vi "add channel to active array_wwarning.vi"(1 "line to add":u32, 2 "line array in":u32[](array[numeric])) -> (0 "line array out":u32[](array[numeric]))   [LabVIEW 2013]
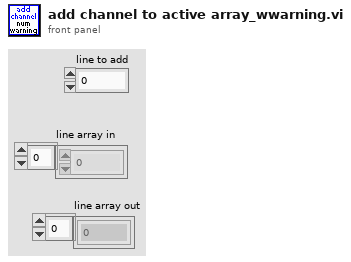
[diagram p1: front panel]
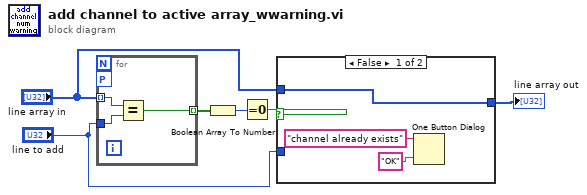
[diagram p0: block diagram]
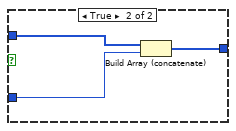
[diagram p2: hidden frame]
diagram:
  n1 = for {
    workers-P: _ -> [_]
    tunnel: "line array in" -> [w8] mode=indexing
    tunnel: "line to add" -> [w9]
    tunnel: [w7] -> w6 mode=indexing
    n2 = Equal?(x=w8, y=w9) -> (x = y?=w7:bool)
  }
  n3 = Boolean Array To Number(Boolean array=w6) -> (number=w5:u32)
  n4 = Equal To 0?(x=w5) -> (x = 0?=w4:bool)
  n5 = case shown="False" w4 {
    tunnel: "line to add" -> [_ w14]
    tunnel: "line array in" -> [w12 w15]
    tunnel: [w12 w13] -> w1
    frame False {
      n6 = One Button Dialog(message="channel already exists", button name ("OK")="OK") -> ()  [unwired: 1 out]
    }
    frame True {
      n7 = Build Array (concatenate)(w15, w14) -> (w13:u32[])
    }
  }
  "line array out" <- w1
